vi "CMD_QUAT2EULER.vi"(6 "Gantry in":refnum<class "Gantry.lvclass">, 8 "error in (no error)":errorcluster, 10 "Arguments":string[](array[string]), 11 "gScript Interpreter in":refnum<class "gScript Interpreter.lvclass">) -> (0 "error out":errorcluster, 3 "gScript Interpreter out":refnum<class "gScript Interpreter.lvclass">, 4 "Gantry out":refnum<class "Gantry.lvclass">)   [LabVIEW 2023, in "gScript Interpreter.lvclass"]
uses:
  gScript Interpreter.lvclass
  Shared Components/Gantry Class/Gantry.lvclass
  Shared Components/Orient3d Class/Orient3d.lvclass
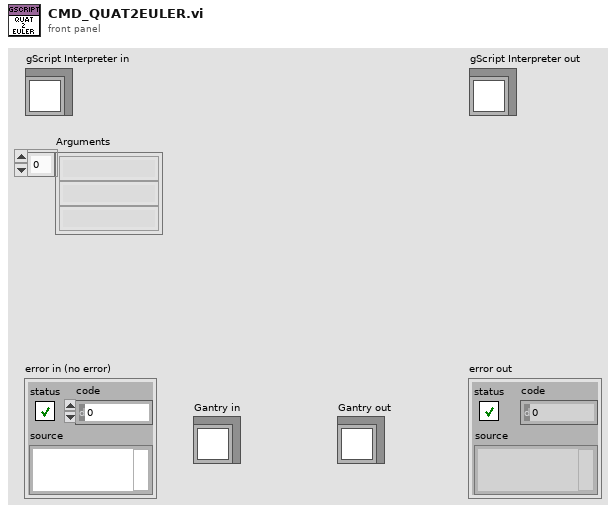
[diagram p1: front panel]
types:
  T1 = typedef "Memory Cell.ctl" = cluster{"type":T2, "x":dbl, "y":dbl, "z":dbl, "w":dbl}
  T2 = typedef "Memory Cell Type Enum.ctl" = enum16{"integer", "float", "vector", "rotation"}
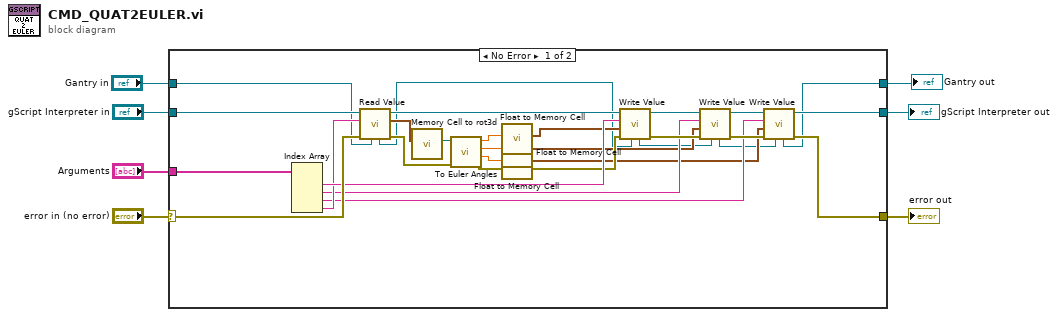
[diagram p0: block diagram]
diagram:
  n1 = case shown="No Error" "error in (no error)" {
    selector: "error in (no error)" -> [w34 w39]
    tunnel: [w18 w39] -> w6
    tunnel: [w13 w38] -> w4
    tunnel: "gScript Interpreter in" -> [w35 w38]
    tunnel: "Arguments" -> [w36 _]
    tunnel: "Gantry in" -> [w12 w37]
    tunnel: [w8 w37] -> w1
    frame No Error {
      n2 = Index Array(array=w36) -> (element #1=w33:string, element #2=w17:string, element #3=w16:string, element #4=w29:string)  [unwired: 4 in]
      n3 = call-dynamic "Read Value.vi"("Gantry in"=w12, "error in (no error)"=w34, "String in"=w29, "gScript Interpreter in"=w35) -> ("error out"=w25:errorcluster, "Memory Cell"=w32:T1, "gScript Interpreter out"=w30:refnum<class "gScript Interpreter.lvclass">, "Gantry out"=w11:refnum<class "Gantry.lvclass">)  [unwired: 4 in]
      n4 = call "Memory Cell to rot3d.vi"("Memory Cell"=w32) -> ("Orient3d out"=w31:refnum<class "Orient3d.lvclass">)  [unwired: 10 in]
      n5 = call "To Euler Angles.vi"("error in"=w25, "Orient3d in"=w31) -> ("error out"=w24:errorcluster, "phi/roll"=w26:dbl, "theta/pitch"=w27:dbl, "psi/yaw"=w28:dbl)  [unwired: 6 in]
      n6 = call "Float to Memory Cell.vi"("Float in"=w28) -> ("Memory Cell"=w23:T1)  [unwired: 10 in]
      n7 = call "Float to Memory Cell.vi"("Float in"=w27) -> ("Memory Cell"=w15:T1)  [unwired: 10 in]
      n8 = call "Float to Memory Cell.vi"("Float in"=w26) -> ("Memory Cell"=w14:T1)  [unwired: 10 in]
      n9 = call-dynamic "Write Value.vi"("Gantry in"=w11, "error in (no error)"=w24, "Value"=w23, "Address"=w33, "gScript Interpreter in"=w30) -> ("error out"=w20:errorcluster, "gScript Interpreter out"=w22:refnum<class "gScript Interpreter.lvclass">, "Gantry out"=w10:refnum<class "Gantry.lvclass">)  [unwired: 4 in]
      n10 = call-dynamic "Write Value.vi"("Gantry in"=w10, "error in (no error)"=w20, "Value"=w15, "Address"=w17, "gScript Interpreter in"=w22) -> ("error out"=w19:errorcluster, "gScript Interpreter out"=w21:refnum<class "gScript Interpreter.lvclass">, "Gantry out"=w9:refnum<class "Gantry.lvclass">)  [unwired: 4 in]
      n11 = call-dynamic "Write Value.vi"("Gantry in"=w9, "error in (no error)"=w19, "Value"=w14, "Address"=w16, "gScript Interpreter in"=w21) -> ("error out"=w18:errorcluster, "gScript Interpreter out"=w13:refnum<class "gScript Interpreter.lvclass">, "Gantry out"=w8:refnum<class "Gantry.lvclass">)  [unwired: 4 in]
    }
    frame Error {
    }
  }
  "error out" <- w6
  "gScript Interpreter out" <- w4
  "Gantry out" <- w1
